vi "maxigauge_get_p.vi"(5 "maxi_delay 3":u32=100, 6 "err_in":errorcluster, 7 "maxi_delay":u32=100, 8 "maxi_delay 2":u32, 9 "?":i32=1, 10 "maxi_visa":refnum<visa-resource-name>="COM8") -> (0 "err_out":errorcluster, 2 "pressure":dbl, 3 "Pressure (Torr)":string)   [LabVIEW 2019]
panel:
  out "read_2":string
  out "read_1":string
  out "Overall Status":bool
  out "Acknowledgement Status":bool
  out "maxi_visa 2":refnum<visa-resource-name>
  in  "maxi_b2r 2":u32
  in  "maxi_b2r":u32
  # "Sensor Number"
  # "VISA"
  # "DELAY"
  # "BYTE AT PORT"
  # "STATUS"
  # "ERROR"
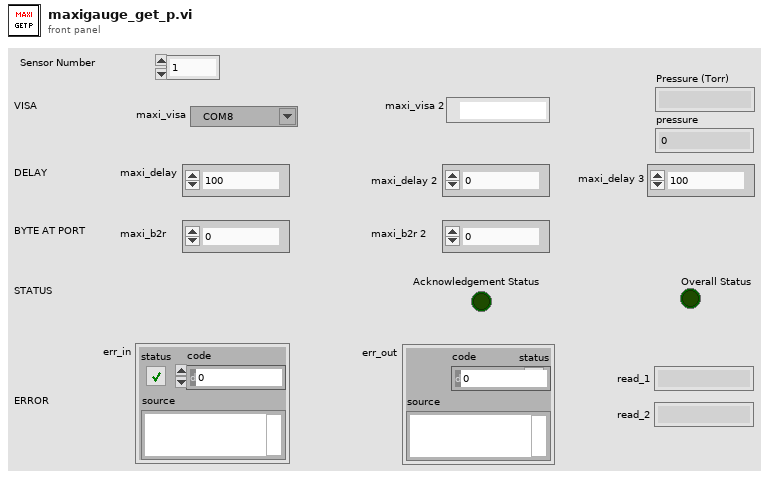
[diagram p1: front panel]
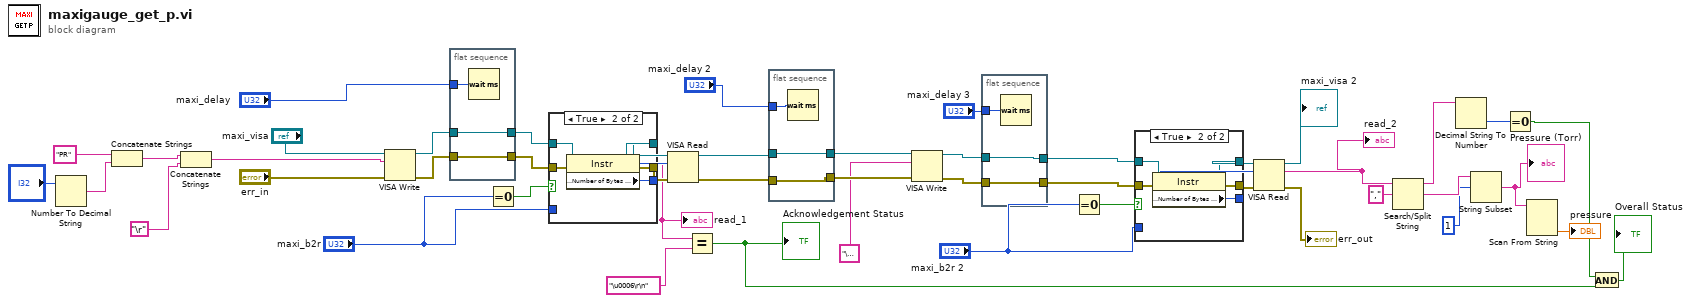
[diagram p0: block diagram]
diagram:
  n1 = Number To Decimal String(number="?") -> (decimal integer string=w4:string)  [unwired: 1 in]
  n2 = Concatenate Strings("PR" ("string"), w4) -> (w5:string)
  n3 = Concatenate Strings(w5, "\r") -> (w21:string)
  n4 = VISA Write(VISA resource name="maxi_visa", write buffer=w21, error in (no error)="err_in") -> (VISA resource name out=w47:refnum<visa-resource-name>, error out=w49:errorcluster)  [unwired: 1 out]
  n5 = flat-sequence {
    tunnel: w49 -> [w51]
    tunnel: [w51] -> w48
    tunnel: w47 -> [w50]
    tunnel: [w50] -> w46
    tunnel: "maxi_delay" -> [w52]
    frame #0 {
      n6 = Wait (ms)(milliseconds to wait=w52) -> ()  [unwired: 1 out]
    }
  }
  n7 = Equal To 0?(x="maxi_b2r") -> (x = 0?=w42:bool)
  n8 = case shown="True" w42 {
    tunnel: w48 -> [w54 w60]
    tunnel: w46 -> [w55 w59]
    tunnel: [w55 w58] -> w40
    tunnel: [w54 w57] -> w39
    tunnel: [w53 w56] -> w38
    tunnel: "maxi_b2r" -> [w53 _]
    frame False {
    }
    frame True {
      n9 = property class="Instr"(reference=w59, error in=w60) -> (reference out=w58:refnum<visa-resource-name>, error out=w57:errorcluster, "Serial Settings:Number of Bytes at Serial Port"=w56:u32)
    }
  }
  n10 = VISA Read(VISA resource name=w40, byte count=w38, error in (no error)=w39) -> (VISA resource name out=w37:refnum<visa-resource-name>, read buffer=w12:string, error out=w36:errorcluster)  [unwired: 1 out]
  "read_1" <- w12
  n11 = Equal?(x=w12, y="\u0006\r\n") -> (x = y?=w8:bool)
  "Acknowledgement Status" <- w8
  n12 = flat-sequence {
    tunnel: [w61] -> w34
    tunnel: w37 -> [w63]
    tunnel: [w63] -> w35
    tunnel: "maxi_delay 2" -> [w62]
    tunnel: w36 -> [w61]
    frame #0 {
      n13 = Wait (ms)(milliseconds to wait=w62) -> ()  [unwired: 1 out]
    }
  }
  n14 = VISA Write(VISA resource name=w35, write buffer="\u0005", error in (no error)=w34) -> (VISA resource name out=w27:refnum<visa-resource-name>, error out=w26:errorcluster)  [unwired: 1 out]
  n15 = flat-sequence {
    tunnel: [w65] -> w33
    tunnel: [w66] -> w32
    tunnel: w27 -> [w66]
    tunnel: w26 -> [w65]
    tunnel: "maxi_delay 3" -> [w64]
    frame #0 {
      n16 = Wait (ms)(milliseconds to wait=w64) -> ()  [unwired: 1 out]
    }
  }
  n17 = Equal To 0?(x="maxi_b2r 2") -> (x = 0?=w31:bool)
  n18 = case shown="True" w31 {
    tunnel: w33 -> [w68 w74]
    tunnel: w32 -> [w69 w73]
    tunnel: [w69 w72] -> w30
    tunnel: [w68 w71] -> w29
    tunnel: [w67 w70] -> w28
    tunnel: "maxi_b2r 2" -> [w67 _]
    frame False {
    }
    frame True {
      n19 = property class="Instr"(reference=w73, error in=w74) -> (reference out=w72:refnum<visa-resource-name>, error out=w71:errorcluster, "Serial Settings:Number of Bytes at Serial Port"=w70:u32)
    }
  }
  n20 = VISA Read(VISA resource name=w30, byte count=w28, error in (no error)=w29) -> (VISA resource name out=→"maxi_visa 2":refnum<visa-resource-name>, read buffer=w19:string, error out=→"err_out":errorcluster)  [unwired: 1 out]
  "read_2" <- w19
  n21 = Search/Split String(string=w19, search string/char (-)=",") -> (substring before match=w15:string, match + rest of string=w17:string)  [unwired: 1 in, 1 out]
  n22 = Decimal String To Number(string=w15) -> (number=w14:i32)  [unwired: 2 in, 1 out]
  n23 = String Subset(string=w17, offset (0)=1) -> (substring=w2:string)  [unwired: 1 in]
  "Pressure (Torr)" <- w2
  n24 = Equal To 0?(x=w14) -> (x = 0?=w9:bool)
  n25 = Scan From String(input string=w2) -> (output 1=→"pressure":dbl)  [unwired: 4 in, 3 out]
  n26 = And(x=w9, y=w8) -> (x .and. y?=→"Overall Status":bool)
